vi "Homing.vi"(10 "error in":errorcluster) -> (2 "error out":errorcluster)   [LabVIEW 2022 SP3]
uses:
  Newport.XPS.CommandInterface
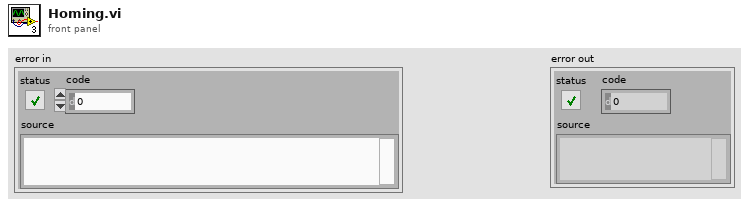
[diagram p1: front panel]
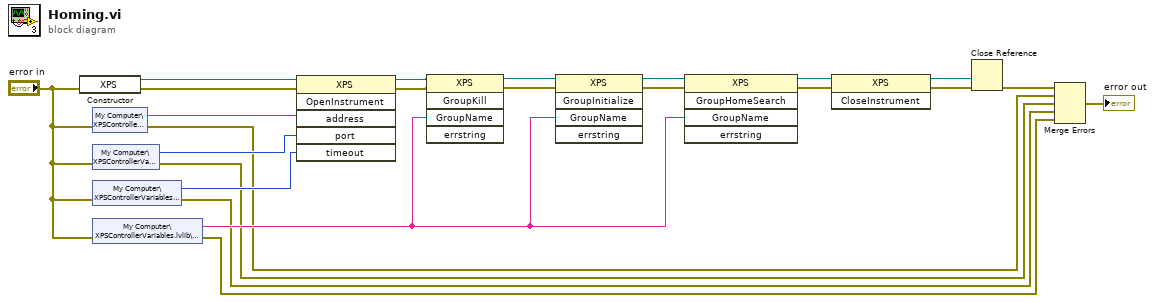
[diagram p0: block diagram]
diagram:
  n1 = constructor class="XPS"(error in="error in") -> (reference out=w22:refnum<k24>, error out=w23:errorcluster)  [unwired: 2 in, 1 out]
  n2 = shared-variable "My Computer\\XPSControllerVariables.lvlib\\IP"(error in="error in") -> (w10:string, error out=w5:errorcluster)
  n3 = shared-variable "My Computer\\XPSControllerVariables.lvlib\\Port"(error in="error in") -> (w9:i16, error out=w4:errorcluster)
  n4 = shared-variable "My Computer\\XPSControllerVariables.lvlib\\Timeout"(error in="error in") -> (w8:i16, error out=w3:errorcluster)
  n5 = shared-variable "My Computer\\XPSControllerVariables.lvlib\\GroupName"(error in="error in") -> (w7:string, error out=w2:errorcluster)
  n6 = invoke class="XPS" method="OpenInstrument"(reference=w22, error in=w23, "address"=w10, "port"=w9, "timeout"=w8) -> (reference out=w15:refnum<k24>, error out=w14:errorcluster)  [unwired: 1 in, 4 out]
  n7 = invoke class="XPS" method="GroupKill"(reference=w15, error in=w14, "GroupName"=w7) -> (reference out=w17:refnum<k24>, error out=w16:errorcluster)  [unwired: 2 in, 3 out]
  n8 = invoke class="XPS" method="GroupInitialize"(reference=w17, error in=w16, "GroupName"=w7) -> (reference out=w19:refnum<k24>, error out=w18:errorcluster)  [unwired: 2 in, 3 out]
  n9 = invoke class="XPS" method="GroupHomeSearch"(reference=w19, error in=w18, "GroupName"=w7) -> (reference out=w13:refnum<k24>, error out=w12:errorcluster)  [unwired: 2 in, 3 out]
  n10 = invoke class="XPS" method="CloseInstrument"(reference=w13, error in=w12) -> (reference out=w21:refnum<k24>, error out=w20:errorcluster)  [unwired: 1 in, 1 out]
  n11 = Close Reference(reference=w21, error in (no error)=w20) -> (error out=w6:errorcluster)
  n12 = Merge Errors(w6, w5, w4, w3, w2) -> (→"error out":errorcluster)
